vi "Catagorize Project Files.vi"(7 "Message Chain":string, 8 "error in (no error)":errorcluster {"code" format="Error %.0f"}, 9 "Processed Files in":set{path}(c389), 10 "Project File Path":path, 11 "VIDoc Parser In":refnum<class "VIDoc Parser.lvclass">) -> (0 "error out":errorcluster {"code" format="Error %.0f"}, 1 "Processed Files out":set{path}(c389), 3 "VIDoc Parser Out":refnum<class "VIDoc Parser.lvclass">)   [LabVIEW 2023, in "VIDoc Parsing.lvlib" / "VIDoc Parser.lvclass"]
uses:
  VIDoc Parser.lvclass
  <vilib>/Utility/EditLVProj/Edit LVProj.lvlib
  Project Documentation/Project Documentation.lvclass
  <vilib>/DMC/VIDoc/Framework/UI Interaction/Interface/UI Interaction.lvclass
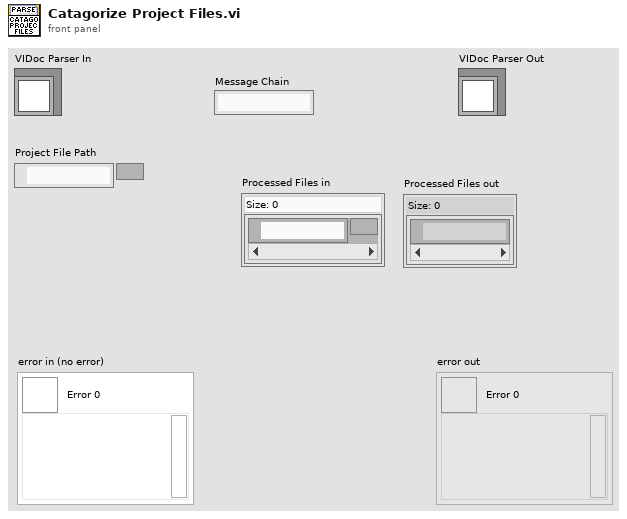
[diagram p1: front panel]
types:
  T1 = typedef "Edit LVProj.lvlib/Library And VI References.ctl" = cluster{"Target Reference":refnum<vi>, "VI References":refnum<vi>[], "Library References":refnum<vi>[]}
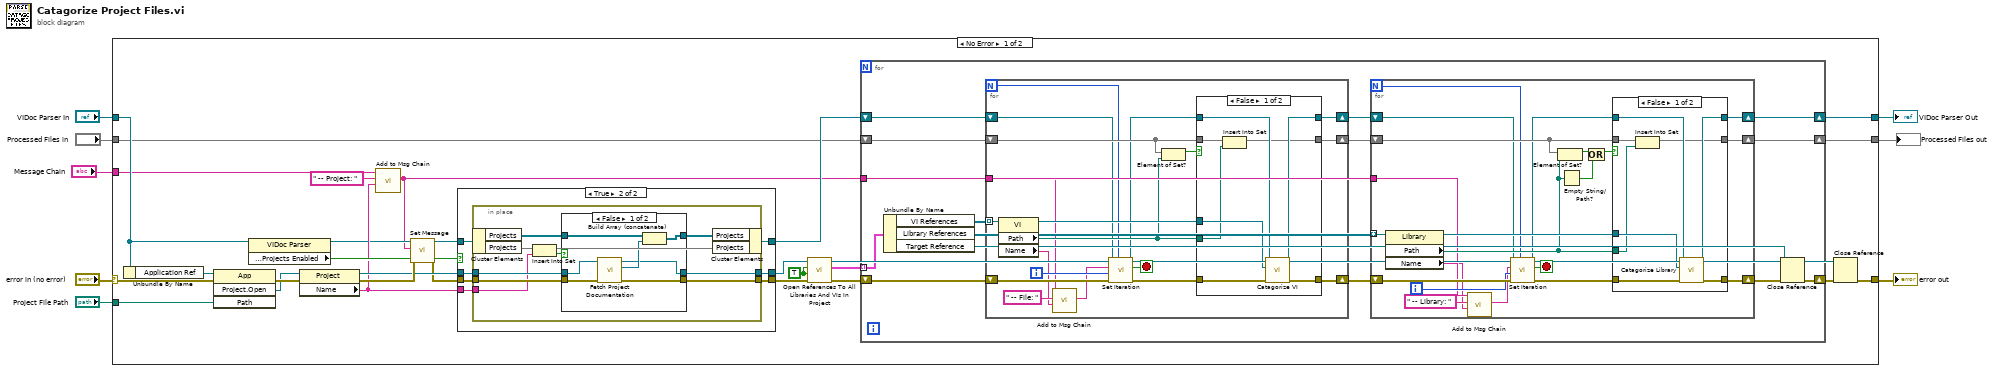
[diagram p0: block diagram]
diagram:
  n1 = case shown="No Error" "error in (no error)" {
    selector: "error in (no error)" -> [w35 w146]
    tunnel: [w20 w146] -> w7
    tunnel: [w29 w145] -> w5
    tunnel: "VIDoc Parser In" -> [w33 w145]
    tunnel: "Project File Path" -> [w34 _]
    tunnel: [w26 w144] -> w3
    tunnel: "Processed Files in" -> [w27 w144]
    tunnel: "Message Chain" -> [w15 _]
    frame No Error {
      w21 = TRUE ("Exclude Targets? (F)")
      n2 = Unbundle By Name(w33) -> ("Application Ref"=w36:refnum<vi>)
      n3 = invoke class="App" method="Project.Open"(reference=w36, error in=w35, "Path"=w34) -> (error out=w25:errorcluster, "Project:Open"=w17:refnum<vi>)  [unwired: 1 in, 2 out]
      n4 = property class="VIDoc Parser"(reference=w33) -> (reference out=w11:refnum<class "VIDoc Parser.lvclass">, "Properties:Enabled:Projects Enabled"=w23:bool)  [unwired: 1 in, 1 out]
      n5 = property class="Project"(reference=w17, error in=w25) -> (reference out=w16:refnum<vi>, error out=w18:errorcluster, "Name"=w13:string)
      n6 = call <vilib>:"Add to Msg Chain.vi"("New"=w13, "Separator (-)"=" -- Project: " ("string"), "Msg Chain in"=w15) -> ("Msg Chain out"=w9:string)  [unwired: 8 in]
      n7 = call "Set Message.vi"("error in (no error)"=w18, "Message"=w9, "VIDoc Parser In"=w11) -> ("error out"=w12:errorcluster, "VIDoc Parser Out"=w10:refnum<class "VIDoc Parser.lvclass">)  [unwired: 7 in]
      n8 = case shown="True" w23 {
        tunnel: [w114 w123] -> w31
        tunnel: w16 -> [w115 w122]
        tunnel: w12 -> [w116 w121]
        tunnel: [w116 w120] -> w24
        tunnel: w10 -> [w114 w119]
        tunnel: [w115 w118] -> w22
        tunnel: w13 -> [_ w117]
        frame False {
        }
        frame True {
          n9 = in-place {
            in-place-border: w122 -> [w125]
            in-place-border: w121 -> [w126]
            in-place-border: [w128] -> w120
            in-place-border: [w127] -> w118
            in-place-border: w117 -> [w124]
            n10 = in-place-cluster #1(w119) -> ("Projects"=w133:refnum<class "Project Documentation.lvclass">[], "Projects"=w131:set{string})
            n11 = Insert Into Set(10:w124, 11:w131) -> (2:w129:bool, 3:w130:set{string})
            n12 = case shown="False" w129 {
              tunnel: w133 -> [w140 w143]
              tunnel: [w139 w143] -> w132
              tunnel: w125 -> [w137 w141]
              tunnel: w126 -> [w136 w142]
              tunnel: [w135 w142] -> w128
              tunnel: [w134 w141] -> w127
              frame False {
                n13 = call "Fetch Project Documentation.vi"("error in (no error)"=w136, "Project in"=w137) -> ("error out"=w135:errorcluster, "Project Doc out"=w138:refnum<class "Project Documentation.lvclass">, "Project out"=w134:refnum<vi>)  [unwired: 7 in]
                n14 = Build Array (concatenate)(w140, w138) -> (w139:refnum<class "Project Documentation.lvclass">[])
              }
              frame True {
              }
            }
            n15 = in-place-cluster #1("Projects"=w132, "Projects"=w130) -> (w123:refnum<class "VIDoc Parser.lvclass">)
          }
        }
      }
      n16 = call <vilib>:"Open References To All Libraries And VIs In Project.vi"("error in (no error)"=w24, "Exclude Targets? (F)"=w21, "Exclude Dependencies? (T)"=w21, "Project in"=w22) -> ("error out"=w32:errorcluster, "VI and Library References"=w30:T1[], "Project out"=w19:refnum<vi>)  [unwired: 5 in]
      n17 = for {
        tunnel: w30 -> [w49] mode=indexing
        shift-right: [w39] -> w28
        shift-left: w32 -> [w51]
        shift-right: [w46] -> w29
        shift-left: w31 -> [w50]
        shift-right: [w40] -> w26
        shift-left: w27 -> [w42]
        tunnel: w9 -> [w37]
        n18 = Unbundle By Name(w49) -> ("VI References"=w48:refnum<vi>[], "Library References"=w43:refnum<vi>[], "Target Reference"=w38:refnum<vi>)
        n19 = for {
          N -> [w90]
          shift-right: [w101] -> w45
          shift-left: w51 -> [w102]
          shift-right: [w100] -> w47
          shift-left: w50 -> [w92]
          tunnel: w48 -> [w99] mode=indexing
          shift-right: [w97] -> w41
          shift-left: w42 -> [w96]
          tunnel: w37 -> [w85]
          i -> [w89]
          stop <- w84 stop-if-true
          n20 = property class="VI"(reference=w99) -> (reference out=w98:refnum<vi>, "Path"=w95:path, "Name"=w87:string)  [unwired: 1 in, 1 out]
          n21 = call <vilib>:"Add to Msg Chain.vi"("New"=w87, "Separator (-)"=" -- File: " ("string"), "Msg Chain in"=w85) -> ("Msg Chain out"=w86:string)  [unwired: 8 in]
          n22 = call "Set Iteration.vi"("Progress Max"=w90, "error in (no error)"=w102, "Progress Value"=w89, "Message (No Message Update)"=w86, "VIDoc Parser In"=w92) -> ("error out"=w93:errorcluster, "Abort?"=w84:bool, "VIDoc Parser Out"=w91:refnum<class "VIDoc Parser.lvclass">)  [unwired: 4 in]
          n23 = Element of Set?(10:w95, 11:w96) -> (3:w94:bool)
          n24 = case shown="False" w94 {
            tunnel: w93 -> [w110 w111]
            tunnel: [w109 w111] -> w101
            tunnel: w91 -> [w108 w112]
            tunnel: [w107 w112] -> w100
            tunnel: w98 -> [w106 _]
            tunnel: [w105 w113] -> w97
            tunnel: w96 -> [w104 w113]
            tunnel: w95 -> [w103 _]
            frame False {
              n25 = Insert Into Set(10:w103, 11:w104) -> (3:w105:set{path})  [unwired: 1 out]
              n26 = call "Catagorize VI.vi"("error in (no error)"=w110, "VI Reference"=w106, "VIDoc Parser In"=w108) -> ("error out"=w109:errorcluster, "VIDoc Parser Out"=w107:refnum<class "VIDoc Parser.lvclass">)  [unwired: 7 in]
            }
            frame True {
            }
          }
        }
        n27 = for {
          N -> [w58]
          shift-right: [w71] -> w44
          shift-left: w45 -> [w72]
          shift-right: [w70] -> w46
          shift-left: w47 -> [w60]
          tunnel: w43 -> [w69] mode=indexing
          shift-right: [w67] -> w40
          shift-left: w41 -> [w66]
          tunnel: w37 -> [w54]
          i -> [w57]
          stop <- w56 stop-if-true
          n28 = property class="Library"(reference=w69) -> (reference out=w68:refnum<vi>, "Path"=w63:path, "Name"=w53:string)  [unwired: 1 in, 1 out]
          n29 = call <vilib>:"Add to Msg Chain.vi"("New"=w53, "Separator (-)"=" -- Library: " ("string"), "Msg Chain in"=w54) -> ("Msg Chain out"=w52:string)  [unwired: 8 in]
          n30 = call "Set Iteration.vi"("Progress Max"=w58, "error in (no error)"=w72, "Progress Value"=w57, "Message (No Message Update)"=w52, "VIDoc Parser In"=w60) -> ("error out"=w61:errorcluster, "Abort?"=w56:bool, "VIDoc Parser Out"=w59:refnum<class "VIDoc Parser.lvclass">)  [unwired: 4 in]
          n31 = Element of Set?(10:w63, 11:w66) -> (3:w65:bool)
          n32 = Empty String/Path?(string/path=w63) -> (empty?=w62:bool)
          n33 = Or(x=w65, y=w62) -> (x .or. y?=w64:bool)
          n34 = case shown="False" w64 {
            tunnel: w61 -> [w80 w81]
            tunnel: [w79 w81] -> w71
            tunnel: w59 -> [w78 w82]
            tunnel: [w77 w82] -> w70
            tunnel: w68 -> [w76 _]
            tunnel: [w75 w83] -> w67
            tunnel: w66 -> [w74 w83]
            tunnel: w63 -> [w73 _]
            frame False {
              n35 = Insert Into Set(10:w73, 11:w74) -> (3:w75:set{path})  [unwired: 1 out]
              n36 = call "Catagorize Library.vi"("error in (no error)"=w80, "Library"=w76, "VIDoc Parser In"=w78) -> ("error out"=w79:errorcluster, "VIDoc Parser Out"=w77:refnum<class "VIDoc Parser.lvclass">)  [unwired: 6 in, 1 out]
            }
            frame True {
            }
          }
        }
        n37 = Close Reference(reference=w38, error in (no error)=w44) -> (error out=w39:errorcluster)
      }
      n38 = Close Reference(reference=w19, error in (no error)=w28) -> (error out=w20:errorcluster)
    }
    frame Error {
    }
  }
  "error out" <- w7
  "VIDoc Parser Out" <- w5
  "Processed Files out" <- w3
